vi "byte array to u8.vi"(1 "索引":i32, 2 "unsigned byte array":u8[](array[numeric])) -> (0 "?":u8)   [LabVIEW 2018]
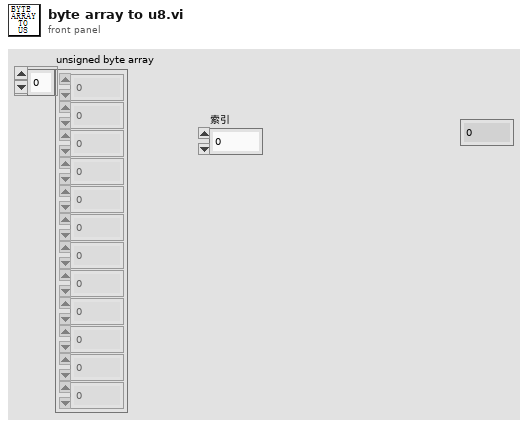
[diagram p1: front panel]
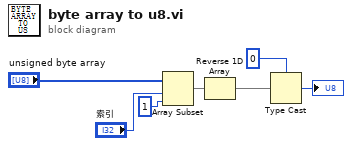
[diagram p0: block diagram]
diagram:
  n1 = Array Subset(array="unsigned byte array", index="索引", length=1 ("长度")) -> (w7:u8[])
  n2 = Reverse 1D Array(array=w7) -> (reversed array=w1:u8[])
  n3 = Type Cast(type=u8 0, x=w1) -> (*(type *) &x=→"?":u8)
